vi "PWRConfigSettings.vi"(0 "PWR In":refnum<visa-resource-name>, 1 "Channel":string="1", 2 "OVP (V)":dbl, 3 "Voltage (V)":dbl, 4 "Current (A)":dbl, 5 "error in (no error)":errorcluster {"code" format="%.0x"}, 6 "PWRID":u8) -> (14 "PWR Out":refnum<visa-resource-name>, 19 "error out":errorcluster)   [LabVIEW 2015]
uses:
  <instrlib>/Agilent N6700 Series/Agilent N6700 Series.lvlib
  <instrlib>/Agilent N87XX Series/Agilent N87XX Series.lvlib
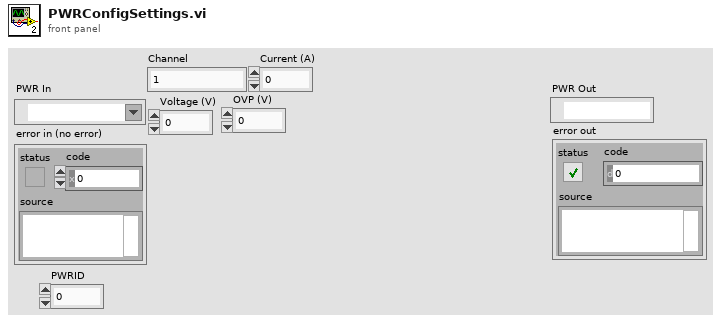
[diagram p1: front panel]
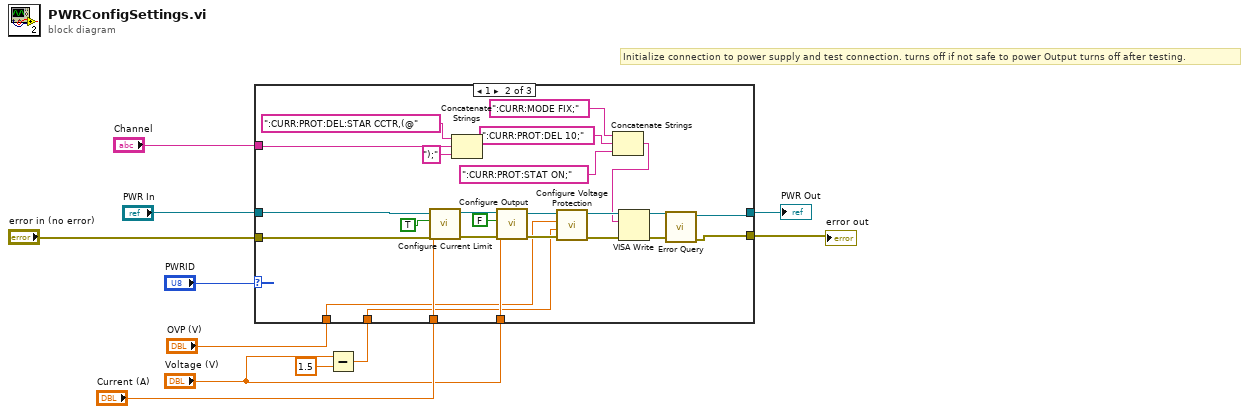
[diagram p0: block diagram]
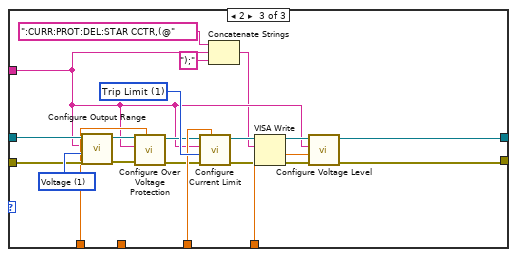
[diagram p3: hidden frame]
diagram:
  # "Initialize connection to power supply and test connection. turns off if not safe to power Output turns off after testing."
  n1 = Subtract(x="Voltage (V)", y=1.5) -> (x-y=w1:dbl)
  n2 = case shown="1" "PWRID" {
    tunnel: "Current (A)" -> [_ w37 w55]
    tunnel: "Voltage (V)" -> [_ w33 w54]
    tunnel: [w13 w15 w40] -> w11
    tunnel: [w12 w14 w39] -> w10
    tunnel: "PWR In" -> [w13 w31 w58]
    tunnel: "error in (no error)" -> [w12 w32 w57]
    tunnel: "OVP (V)" -> [_ w27 w45]
    tunnel: "Channel" -> [_ w24 w43]
    tunnel: w1 -> [_ w28 _]
    frame 0, Default {
    }
    frame 1 {
      n3 = call <instrlib>:"Configure Current Limit.vi"("error in (no error)"=w32, "Current Limit (0.0 A)"=w37, "Enable Current Protection (F: Disable)"=TRUE, "VISA resource name"=w31) -> ("error out"=w35:errorcluster, "VISA resource name out"=w36:refnum<visa-resource-name>)  [unwired: 6 in]
      n4 = Concatenate Strings(":CURR:PROT:DEL:STAR CCTR,(@" ("format string"), w24, ");" ("string")) -> ()  [unwired: 1 out]
      n5 = call <instrlib>:"Configure Output.vi"("error in (no error)"=w35, "Voltage Level (0.0 V)"=w33, "Enable Output (T: Enable)"=FALSE, "VISA resource name"=w36) -> ("error out"=w30:errorcluster, "VISA resource name out"=w29:refnum<visa-resource-name>)  [unwired: 6 in]
      n6 = call <instrlib>:"Configure Voltage Protection.vi"("error in (no error)"=w30, "Under-Voltage Protection (0.0 V)"=w28, "Over-Voltage Protection (5.0 V)"=w27, "VISA resource name"=w29) -> ("error out"=w22:errorcluster, "VISA resource name out"=w23:refnum<visa-resource-name>)  [unwired: 6 in]
      n7 = Concatenate Strings(":CURR:MODE FIX;" ("string"), ":CURR:PROT:DEL 10;" ("write buffer"), ":CURR:PROT:STAT ON;" ("write buffer")) -> (w19:string)
      n8 = VISA Write(VISA resource name=w23, write buffer=w19, error in (no error)=w22) -> (VISA resource name out=w17:refnum<visa-resource-name>, error out=w16:errorcluster)  [unwired: 1 out]
      n9 = call <instrlib>:"Error Query.vi"("error in (no error)"=w16, "VISA resource name"=w17) -> ("error out"=w14:errorcluster, "VISA resource name out"=w15:refnum<visa-resource-name>)  [unwired: 6 in, 2 out]
    }
    frame 2 {
      w56 = 1 items=["Regulatory Limit", "Trip Limit"] ("Behavior (0: Regulatory Limit)")
      w59 = 1 items=["Voltage"=1, "Current"=0] ("Range Type (1: Voltage)")
      n10 = call <instrlib>:"Configure Output Range.vi"("error in (no error)"=w57, "Range Type (1: Voltage)"=w59, "Channel Name (1)"=w43, "VISA resource name"=w58) -> ("error out"=w52:errorcluster, "VISA resource name out"=w53:refnum<visa-resource-name>)  [unwired: 6 in]
      n11 = call <instrlib>:"Configure Over Voltage Protection.vi"("Limit (0.0 volts)"=w45, "error in (no error)"=w52, "Channel Name (1)"=w43, "VISA resource name"=w53) -> ("error out"=w50:errorcluster, "VISA resource name out"=w51:refnum<visa-resource-name>)  [unwired: 6 in]
      n12 = call <instrlib>:"Configure Current Limit.vi"("Limit (0.0 amps)"=w55, "error in (no error)"=w50, "Behavior (0: Regulatory Limit)"=w56, "Channel Name (1)"=w43, "VISA resource name"=w51) -> ("error out"=w48:errorcluster, "VISA resource name out"=w49:refnum<visa-resource-name>)  [unwired: 5 in]
      n13 = Concatenate Strings(":CURR:PROT:DEL:STAR CCTR,(@" ("format string"), w43, ");" ("string")) -> (w41:string)
      n14 = VISA Write(VISA resource name=w49, write buffer=w41, error in (no error)=w48) -> (VISA resource name out=w47:refnum<visa-resource-name>, error out=w46:errorcluster)  [unwired: 1 out]
      n15 = call <instrlib>:"Configure Voltage Level.vi"("error in (no error)"=w46, "Level  (0.0 volts)"=w54, "Channel Name (1)"=w43, "VISA resource name"=w47) -> ("error out"=w39:errorcluster, "VISA resource name out"=w40:refnum<visa-resource-name>)  [unwired: 6 in]
    }
  }
  "PWR Out" <- w11
  "error out" <- w10
